vi "Clear-reference.vi"(8 "error in (no error)":errorcluster, 10 "Panes reference":T1) -> (0 "error out":errorcluster, 3 "Panes out":refnum<class "Panes.lvclass">)   [LabVIEW 2013, in "PaneToggle.lvlib" / "Panes.lvclass"]
uses:
  Panes.lvclass
  Object-reference.ctl
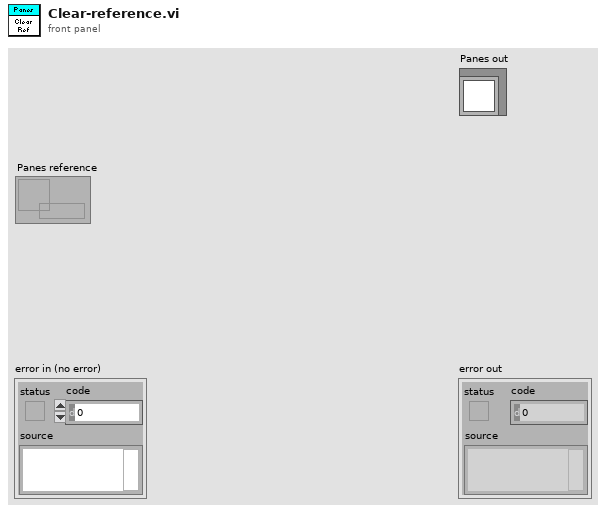
[diagram p1: front panel]
types:
  T1 = typedef "PaneToggle.lvlib/Panes.lvclass/Object-reference.ctl" = refnum<data-value>
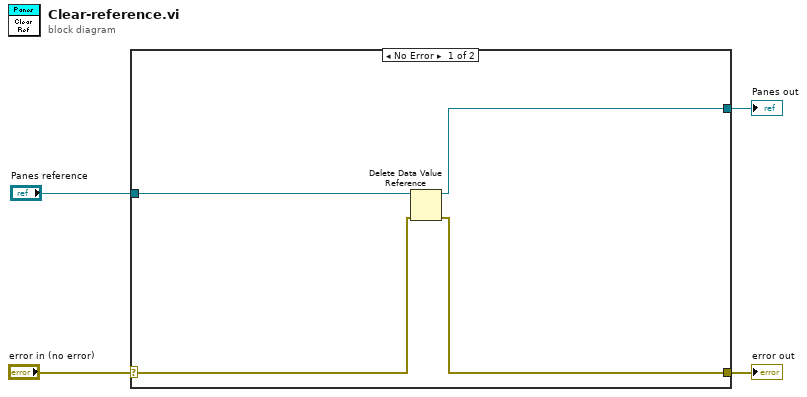
[diagram p0: block diagram]
diagram:
  n1 = case shown="No Error" "error in (no error)" {
    selector: "error in (no error)" -> [w7 w9]
    tunnel: [w6 w9] -> w3
    tunnel: [w5 _] -> w2
    tunnel: "Panes reference" -> [w8 _]
    frame No Error {
      n2 = Delete Data Value Reference(data value reference=w8, error in=w7) -> (data value=w5:refnum<class "Panes.lvclass">, error out=w6:errorcluster)
    }
    frame Error {
    }
  }
  "error out" <- w3
  "Panes out" <- w2
